vi "GRIMMMeasurementGFV.vi"(8 "error in (no error)":errorcluster, 10 "Variant in":variant, 11 "GRIMMMeasEnum":T1=enum."InsertMeasurement") -> (0 "error out":errorcluster, 3 "Variant out":variant)   [LabVIEW 2013]
doc: "Use this template to build a VI to use as a subVI."
uses:
  GRIMMmeasurementEnum.ctl
  GRIMMmeasurementCluster.ctl
panel:
  out "element 4":dbl
  out "element 3":dbl
  out "element 2":dbl
  out "element":dbl
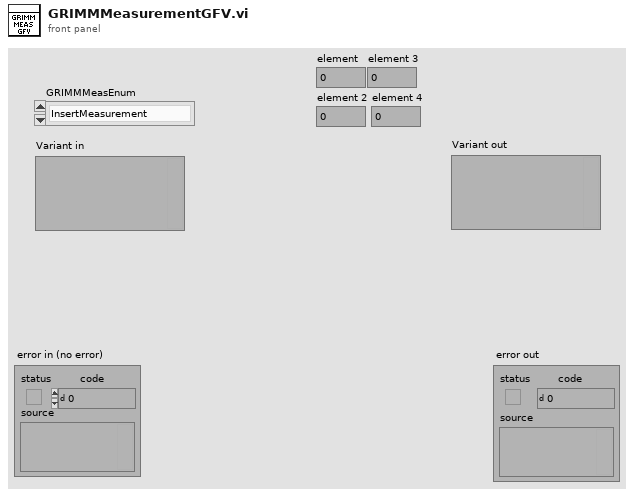
[diagram p1: front panel]
types:
  T1 = typedef "GRIMMmeasurementEnum.ctl" = enum16{"Get CountVsDiameter", "Get CountsVsTime", "Get Raw Data", "InsertMeasurement", "Init"}
  T2 = typedef "GRIMMmeasurementCluster.ctl" = cluster{"Threshold Bin size":dbl[], "Measurement Data":i32[]}
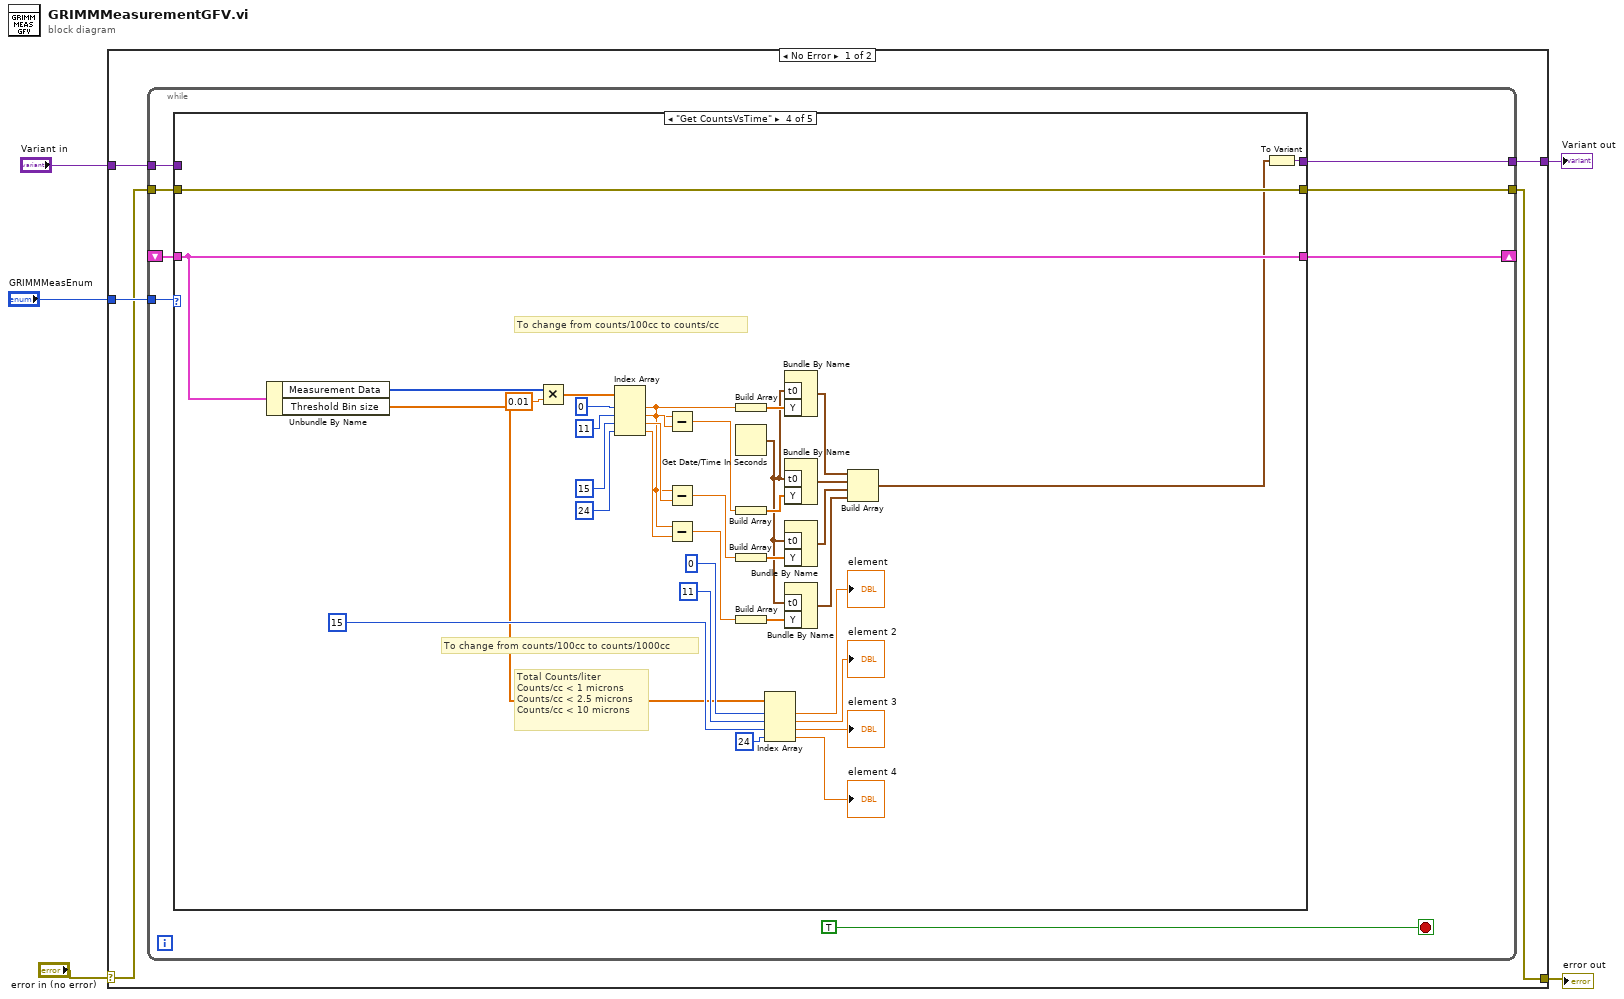
[diagram p0: block diagram]
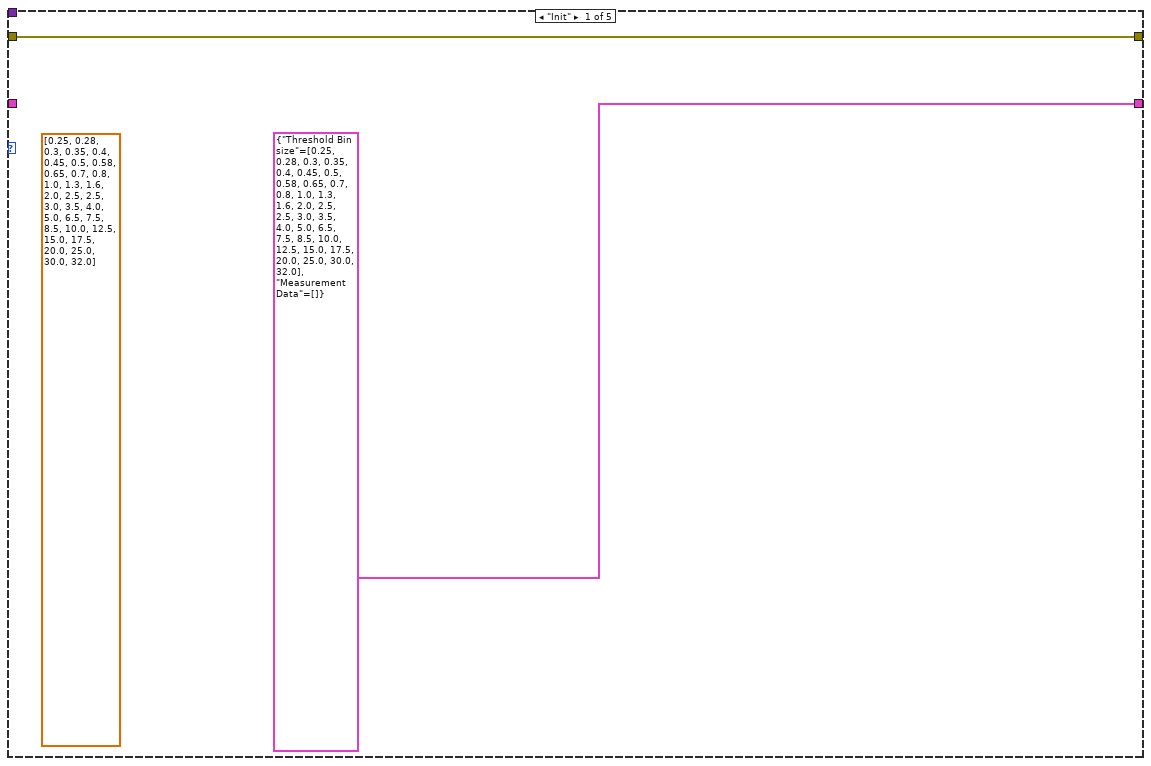
[diagram p2: hidden frame]
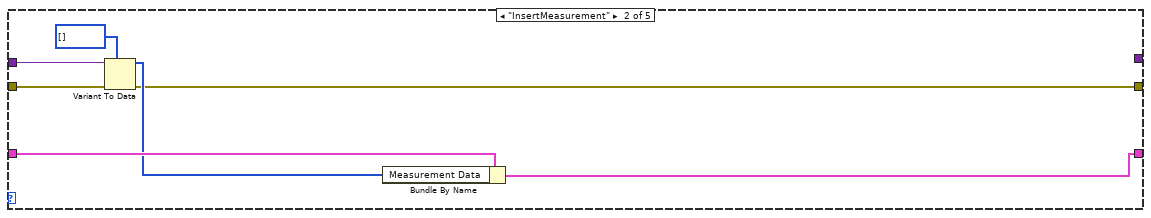
[diagram p3: hidden frame]
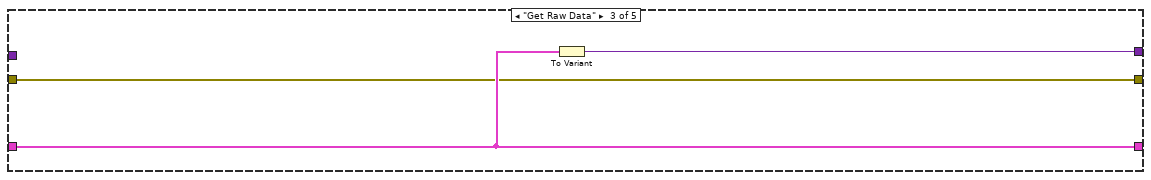
[diagram p4: hidden frame]
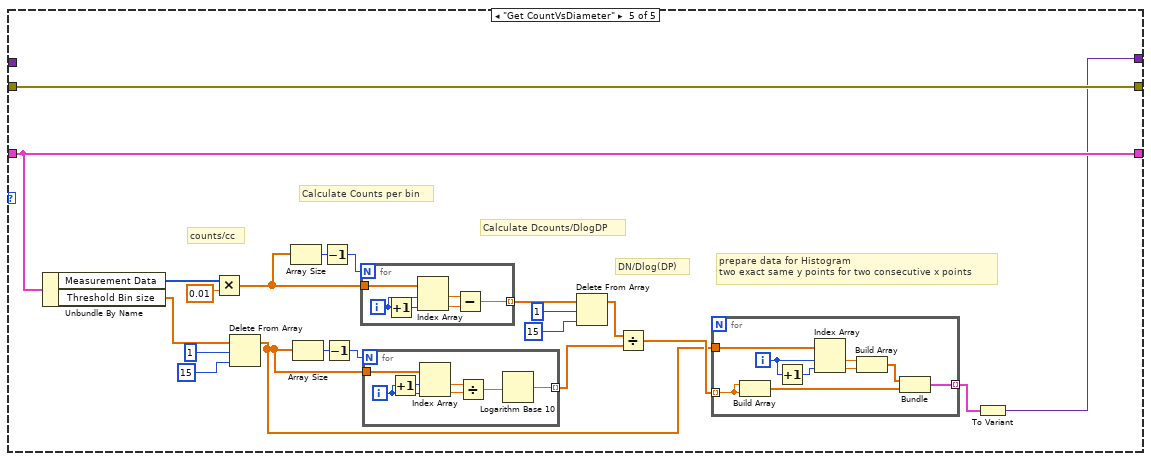
[diagram p5: hidden frame]
diagram:
  n1 = case shown="No Error" "error in (no error)" {
    selector: "error in (no error)" -> [w8 w111]
    tunnel: [w7 w111] -> w4
    tunnel: "GRIMMMeasEnum" -> [w10 _]
    tunnel: "Variant in" -> [w9 w110]
    tunnel: [w6 w110] -> w1
    frame No Error {
      n2 = while {
        tunnel: w10 -> [w17]
        shift-right: [w16] -> _
        shift-left: _ -> [w15]
        tunnel: w9 -> [w14]
        tunnel: w8 -> [w13]
        tunnel: [w12] -> w7
        tunnel: [w11] -> w6
        stop <- TRUE stop-if-true
        n3 = case shown="\"Get CountsVsTime\"" w17 {
          tunnel: [T2 {"Threshold Bin size"=[0.25, 0.28, 0.3, 0.35, 0.4, 0.45, 0.5, 0.58, 0.65, 0.7, 0.8, 1.0, 1.3, 1.6, 2.0, 2.5, 2.5, 3.0, 3.5, 4.0, 5.0, 6.5, 7.5, 8.5, 10.0, 12.5, 15.0, 17.5, 20.0, 25.0, 30.0, 32.0], "Measurement Data"=[]} w26 w30 w64 w86] -> w16
          tunnel: w15 -> [_ w27 w30 w64 w86]
          tunnel: w14 -> [_ w24 _ _ _]
          tunnel: w13 -> [w20 w25 w28 w65 w87]
          tunnel: [w20 w21 w28 w65 w87] -> w12
          tunnel: [_ _ w29 w66 w67] -> w11
          frame "Init" {
            (unwired) dbl[] [0.25, 0.28, 0.3, 0.35, 0.4, 0.45, 0.5, 0.58, 0.65, 0.7, 0.8, 1.0, 1.3, 1.6, 2.0, 2.5, 2.5, 3.0, 3.5, 4.0, 5.0, 6.5, 7.5, 8.5, 10.0, 12.5, 15.0, 17.5, 20.0, 25.0, 30.0, 32.0] ("Threshold Bin size")
          }
          frame "InsertMeasurement" {
            n4 = Variant To Data(error in=w25, type=i32[] [] ("f"), Variant=w24) -> (data=w22:i32[], error out=w21:errorcluster)
            n5 = Bundle By Name(cluster=w27, "Measurement Data"=w22) -> (w26:T2)
          }
          frame "Get Raw Data" {
            n6 = To Variant(anything=w30) -> (Variant=w29:variant)
          }
          frame "Get CountsVsTime" {
            # "To change from counts/100cc to counts/1000cc"
            # "To change from counts/100cc to counts/cc"
            # "Total Counts/liter\nCounts/cc < 1 microns\nCounts/cc < 2.5 microns\nCounts/cc < 10 microns"
            n7 = Unbundle By Name(w64) -> ("Measurement Data"=w63:i32[], "Threshold Bin size"=w52:dbl[])
            n8 = Multiply(x=w63, y=0.01) -> (x*y=w61:dbl[])
            n9 = Index Array(array=w61, index #1=0 ("index"), index #2=11 ("index"), index #3=15 ("index"), index #4=24 ("index")) -> (element #1=w44:dbl, element #2=w47:dbl, element #3=w46:dbl, element #4=w45:dbl)
            n10 = Subtract(x=w44, y=w47) -> (x-y=w37:dbl)
            n11 = Subtract(x=w44, y=w46) -> (x-y=w36:dbl)
            n12 = Subtract(x=w44, y=w45) -> (x-y=w35:dbl)
            n13 = Build Array(w44) -> (w43:dbl[])
            n14 = Get Date/Time In Seconds() -> (seconds since 1Jan1904=w31:timestamp)
            n15 = Build Array(w37) -> (w40:dbl[])
            n16 = Build Array(w36) -> (w39:dbl[])
            n17 = Build Array(w35) -> (w38:dbl[])
            n18 = Index Array(array=w52, index #1=0 ("index"), index #2=11 ("index"), index #3=15 ("index"), index #4=24 ("index")) -> (element #1=→"element":dbl, element #2=→"element 2":dbl, element #3=→"element 3":dbl, element #4=→"element 4":dbl)
            n19 = Bundle By Name("t0"=w31, "Y"=w43) -> (w41:waveform(dbl))  [unwired: 1 in]
            n20 = Bundle By Name("t0"=w31, "Y"=w40) -> (w34:waveform(dbl))  [unwired: 1 in]
            n21 = Bundle By Name("t0"=w31, "Y"=w39) -> (w33:waveform(dbl))  [unwired: 1 in]
            n22 = Bundle By Name("t0"=w31, "Y"=w38) -> (w32:waveform(dbl))  [unwired: 1 in]
            n23 = Build Array(w41, w34, w33, w32) -> (w42:waveform(dbl)[])
            n24 = To Variant(anything=w42) -> (Variant=w66:variant)
          }
          frame "Get CountVsDiameter" {
            # "counts/cc"
            # "DN/Dlog(DP)"
            # "Calculate Dcounts/DlogDP"
            # "prepare data for Histogram\ntwo exact same y points for two consecutive x points"
            # "Calculate Counts per bin"
            n25 = Unbundle By Name(w86) -> ("Measurement Data"=w74:i32[], "Threshold Bin size"=w78:dbl[])
            n26 = Multiply(x=w74, y=0.01) -> (x*y=w73:dbl[])
            n27 = Delete From Array(array=w78, length=1, index=15) -> (array with subset deleted=w69:dbl[])  [unwired: 1 out]
            n28 = Array Size(array=w73) -> (size(s)=w85:i32)
            n29 = Array Size(array=w69) -> (size(s)=w76:i32)
            n30 = Decrement(x=w85) -> (x-1=w84:i32)
            n31 = Decrement(x=w76) -> (x-1=w77:i32)
            n32 = for {
              N: w84 -> [_]
              tunnel: w73 -> [w109]
              tunnel: [w104] -> w83 mode=indexing
              i -> [w108]
              n33 = Increment(x=w108) -> (x+1=w107:i32)
              n34 = Index Array(array=w109, index #1=w108, index #2=w107) -> (element #1=w105:dbl, element #2=w106:dbl)
              n35 = Subtract(x=w105, y=w106) -> (x-y=w104:dbl)
            }
            n36 = for {
              N: w77 -> [_]
              tunnel: w69 -> [w103]
              tunnel: [w97] -> w71 mode=indexing
              i -> [w102]
              n37 = Increment(x=w102) -> (x+1=w101:i32)
              n38 = Index Array(array=w103, index #1=w101, index #2=w102) -> (element #1=w100:dbl, element #2=w99:dbl)
              n39 = Divide(x=w100, y=w99) -> (x/y=w98:dbl)
              n40 = Logarithm Base 10(1:w98) -> (0:w97:dbl)
            }
            n41 = Delete From Array(array=w83, length=1, index=15) -> (array with subset deleted=w72:dbl[])  [unwired: 1 out]
            n42 = Divide(x=w72, y=w71) -> (x/y=w70:dbl[])
            n43 = for {
              tunnel: w70 -> [w93] mode=indexing
              tunnel: w69 -> [w96]
              tunnel: [w88] -> w68 mode=indexing
              i -> [w95]
              n44 = Build Array(w93, w93) -> (w89:dbl[])
              n45 = Increment(x=w95) -> (x+1=w94:i32)
              n46 = Index Array(array=w96, index #1=w95, index #2=w94) -> (element #1=w92:dbl, element #2=w91:dbl)
              n47 = Build Array(w92, w91) -> (w90:dbl[])
              n48 = Bundle(w90, w89) -> (w88:cluster{dbl[], dbl[]})  [unwired: 1 in]
            }
            n49 = To Variant(anything=w68) -> (Variant=w67:variant)
          }
        }
      }
    }
    frame Error {
    }
  }
  "error out" <- w4
  "Variant out" <- w1
